vi "readFILE.vi"() -> ()   [LabVIEW 2023]
panel:
  in  "stop":bool
  out "text":string
  in  "file path (use dialog)":path
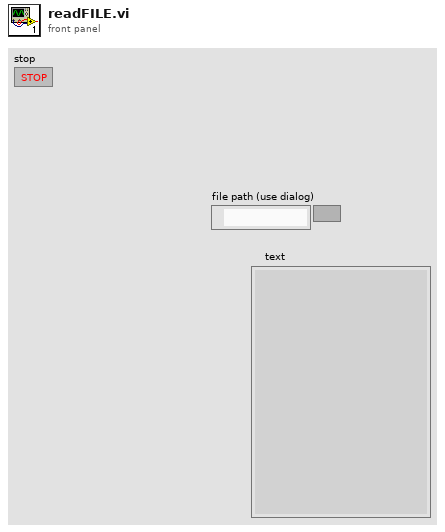
[diagram p1: front panel]
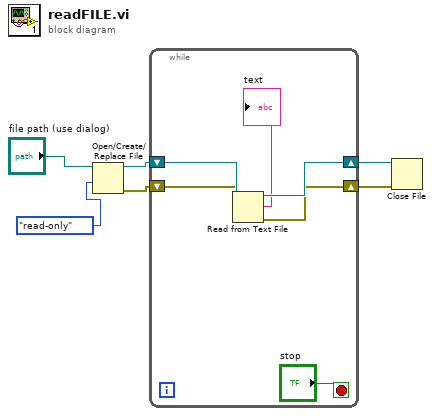
[diagram p0: block diagram]
diagram:
  n1 = Open/Create/Replace File(file path (use dialog)="file path (use dialog)", access (0:read/write)=enum16{"read/write", "read-only", "write-only"}."read-only") -> (refnum out=w5:refnum<file>, error out=w4:errorcluster)  [unwired: 4 in, 1 out]
  n2 = while {
    shift-right: [w10] -> w3
    shift-left: w5 -> [w12]
    shift-right: [w9] -> w2
    shift-left: w4 -> [w11]
    stop <- "stop" stop-if-true
    n3 = Read from Text File(file (use dialog)=w12, error in=w11) -> (refnum out=w10:refnum<file>, text=→"text":string, error out=w9:errorcluster)  [unwired: 2 in, 1 out]
  }
  n4 = Close File(refnum=w3, error in=w2) -> ()  [unwired: 2 out]
